vi "Operator show list with space bar continue.vi"(8 "error in (no error)":errorcluster, 10 "Item Names":string[](array[string]), 11 "Message":string) -> (0 "error out":errorcluster)   [LabVIEW 2013]
uses:
  <vilib>/event_ctls.llb/eventvkey.ctl
panel:
  in  "Listbox":i32(listbox)
  # "Operator Message"
  # "Press SPACE BAR to continue"
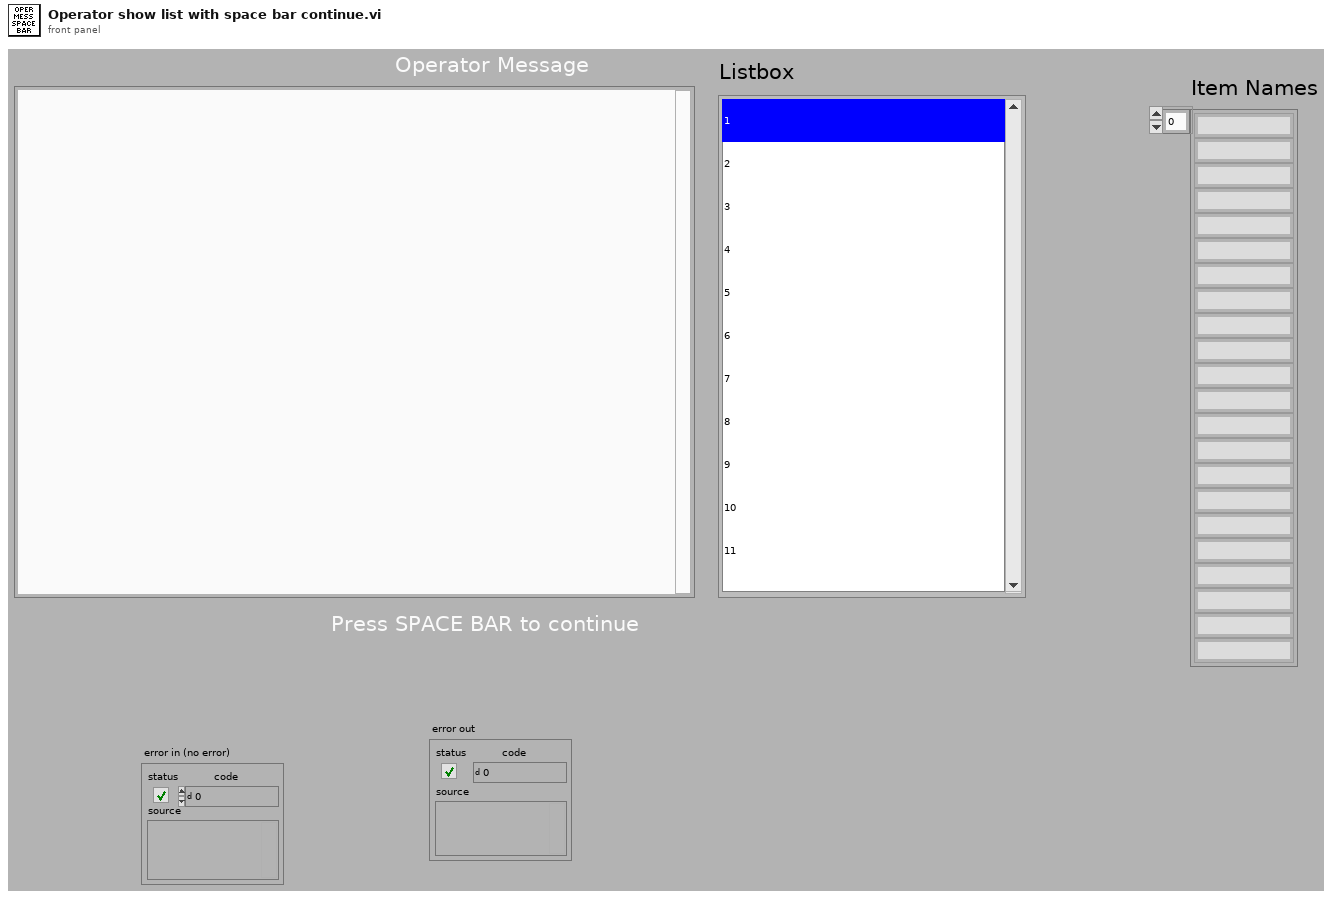
[diagram p1: front panel]
types:
  T1 = typedef "eventvkey.ctl" = enum16{"ASCII", "Enter", "Return", "Shift", "Ctrl", "Alt", "Cmd", "Opt", "Caps", "NumLock", "Clear", "Break", "Up", "Down", "Left", "Right", "Insert", "Delete", "Home", "End", "PageUp", "PageDown", "Escape", "Help", "Pause", "ScrollLock", "F1", "F2", "F3", "F4", "F5", "F6", "F7", "F8", "F9", "F10", "F11", "F12", "F13", "F14", "F15", "F16", "F17", "F18", "F19", "F20", "F21", "F22", "F23", "F24", "Play", "VolumeUp", "VolumeDown", "Mute", "Two Byte Char"}
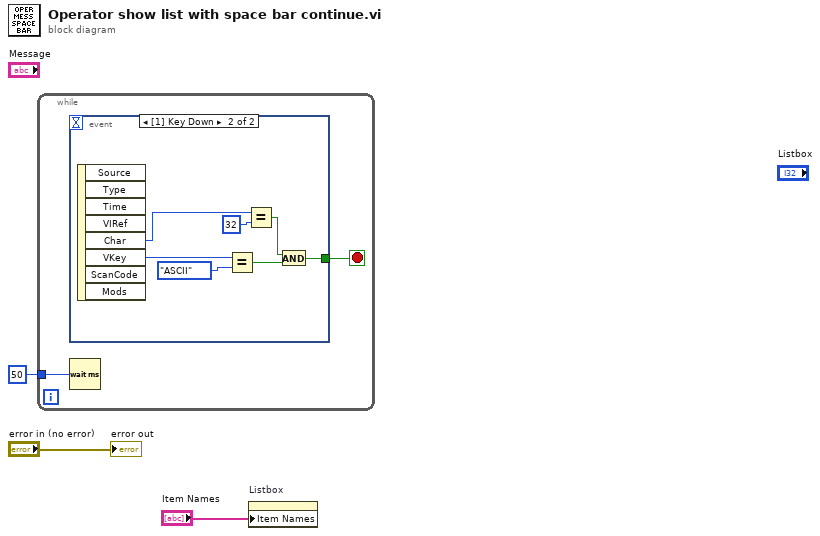
[diagram p0: block diagram]
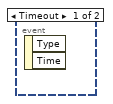
[diagram p2: hidden frame]
diagram:
  n1 = while {
    tunnel: u32 50 ("milliseconds to wait") -> [w5]
    stop <- w4 stop-if-true
    n2 = event shown="[1] Key Down" {
      selector: _ -> [_ _]
      dyn-events: _ -> [_ _]
      timeout: _ -> [_ _]
      tunnel: [_ w6] -> w4
      event Timeout {
        n3 = event-data() -> ()  [unwired: 1 in, 2 out]
      }
      event Key Down {
        n4 = event-data() -> ("Char"=w12:i16, "VKey"=w10:T1)  [unwired: 1 in, 6 out]
        n5 = Equal?(x=w10, y=eventvkey."ASCII" ("VKey")) -> (x = y?=w7:bool)
        n6 = Equal?(x=w12, y=i16 32) -> (x = y?=w8:bool)
        n7 = And(x=w8, y=w7) -> (x .and. y?=w6:bool)
      }
    }
    n8 = Wait (ms)(milliseconds to wait=w5) -> ()  [unwired: 1 out]
  }
  n9 = property on="Listbox" class="LstBox (strict)"("Item Names"="Item Names") -> ()  [unwired: 2 in, 2 out]
  "error out" <- "error in (no error)"
